vi "dsdll_output_write_auto_float32.vi"(5 "volume (1: don't change volume)":i32=1 min=-10000 max=1 step=1, 6 "looped mode (true)":bool=TRUE, 7 "play (true)":bool=TRUE, 8 "error in":errorcluster, 9 "transpose (false)":bool, 10 "float32 samples":sgl[][](array[numeric]), 11 "dsdll instance in":T1={"dsdll path"=path "E:/LVprog/DirectSoundDLL/dsdll.dll", "dsdll handle"=[], "output devices"=[], "capture devices"=[]}) -> (0 "error out":errorcluster, 3 "dsdll instance out":T1)   [LabVIEW 2020, in "dsdll.lvlib"]
doc: "Call this to write sample data into the output device buffer. \nOptionally starts playback and sets volume. If the 'volume' input left unconnectged it does not change the volume. The range of the volume is {-10000 to 0} where -10000 is equal to -100dB and 0 is 0dB (full volume).\nThe 'looped mode' option enables playback of the waveform in an infinite loop. If set to false the waveform will be played just once.\n\n\nData is automatically converted to the needed wave output format from float32, it is also denormalized from <-1;1> range to fullscale. Data is organized as 2D array:\nIf the 'transpose' input is false: rows = channels, columns = samples.\nIf 'transpose' is true: columns = channels; rows = samples."
uses:
  dsdll.lvlib
  dsdll_instance.ctl
  dsdll_device_record.ctl
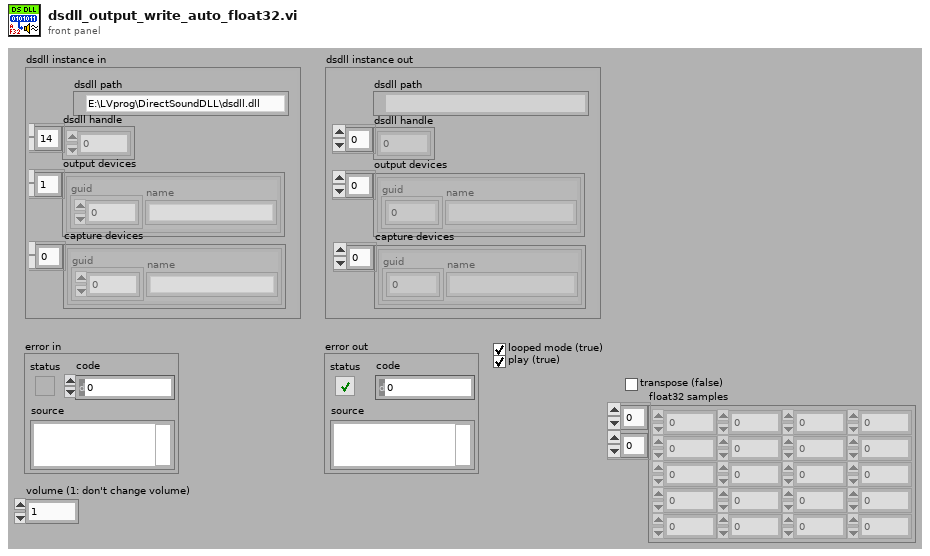
[diagram p1: front panel]
types:
  T1 = typedef "dsdll.lvlib/dsdll_instance.ctl" = cluster{"dsdll path":path, "dsdll handle":u8[], "output devices":T2[], "capture devices":T2[]}
  T2 = typedef "dsdll.lvlib/dsdll_device_record.ctl" = cluster{"guid":u8[], "name":string}
  T3 = typedef "dsdll.lvlib/dsdll_sample_format.ctl" = enum16{"IEEE float 32", "PCM 16 bit"}
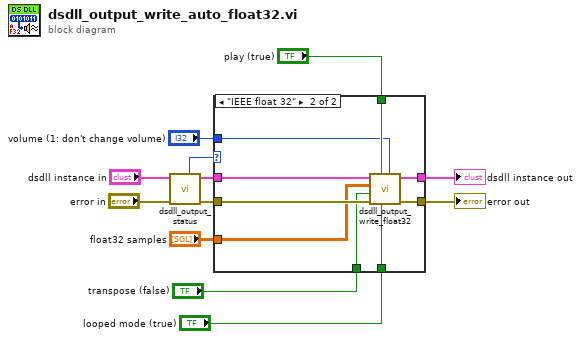
[diagram p0: block diagram]
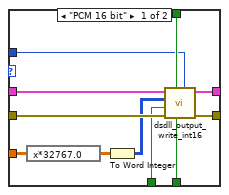
[diagram p2: hidden frame]
diagram:
  n1 = call "dsdll_output_status.vi"("error in"="error in", "dsdll instance in"="dsdll instance in") -> ("error out"=w10:errorcluster, "dsdll instance out"=w9:T1, "format"=w5:T3)  [unwired: 3 in, 4 out]
  n2 = case shown="\"IEEE float 32\"" w5 {
    tunnel: w10 -> [w23 w32]
    tunnel: w9 -> [w22 w31]
    tunnel: [w21 w30] -> w8
    tunnel: [w20 w29] -> w7
    tunnel: "play (true)" -> [w19 w28]
    tunnel: "float32 samples" -> [w18 w26]
    tunnel: "transpose (false)" -> [w16 w27]
    tunnel: "volume (1: don't change volume)" -> [w14 w25]
    tunnel: "looped mode (true)" -> [w13 w24]
    frame "PCM 16 bit" {
      n3 = expression code="x*32767.0"(w18) -> (w15:sgl[][])
      n4 = To Word Integer(number=w15) -> (16bit integer=w17:i16[][])
      n5 = call "dsdll_output_write_int16.vi"("volume (1: don't change volume)"=w14, "looped mode (true)"=w13, "play (true)"=w19, "error in"=w23, "transpose (false)"=w16, "int16 samples"=w17, "dsdll instance in"=w22) -> ("error out"=w21:errorcluster, "dsdll instance out"=w20:T1)  [unwired: 3 in]
    }
    frame "IEEE float 32" {
      n6 = call "dsdll_output_write_float32.vi"("volume (1: don't change volume)"=w25, "looped mode (true)"=w24, "play (true)"=w28, "error in"=w32, "transpose (false)"=w27, "float32 samples"=w26, "dsdll instance in"=w31) -> ("error out"=w30:errorcluster, "dsdll instance out"=w29:T1)  [unwired: 3 in]
    }
  }
  "error out" <- w8
  "dsdll instance out" <- w7
